vi "Read Profile Data From File.vi"(0 "Profile Data File":path=path "C:/Grabit/Software/VI's/Profiles.ini", 5 "Profile Name":string="Profile1", 11 "error in (no error)":errorcluster) -> (4 "Profile Data":string="0001020304050607080910111213141516171819202122232425262728293031323334353637383940414243444546474849", 15 "error out":errorcluster)   [LabVIEW 2015]
uses:
  <vilib>/Utility/config.llb/Read Key (String).vi
  <vilib>/Utility/config.llb/NI_LVConfig.lvlib
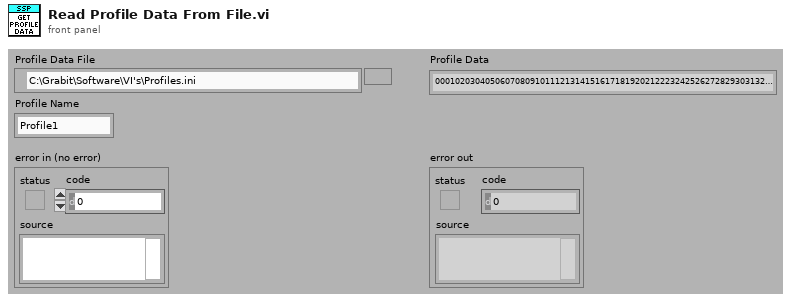
[diagram p1: front panel]
types:
  T1 = typedef "NI_LVConfig.lvlib/Config Data RefNum.ctl" = refnum<k1>
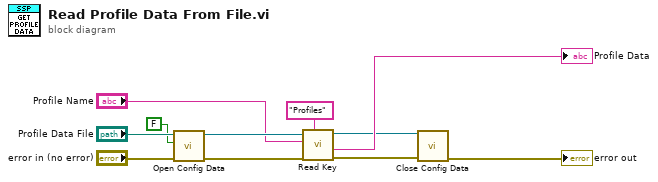
[diagram p0: block diagram]
diagram:
  n1 = call <vilib>:"Open Config Data.vi"("error in (no error)"="error in (no error)", "create file if necessary (T)"=FALSE, "configuration file path"="Profile Data File") -> ("error out"=w10:errorcluster, "refnum"=w11:T1)  [unwired: 6 in, 1 out]
  n2 = call-poly <vilib>:"Read Key.vi"("section"="Profiles", "error in (no error)"=w10, "key"="Profile Name", "refnum"=w11) -> ("error out"=w3:errorcluster, "value"=→"Profile Data":string, "refnum out"=w4:T1)  [unwired: 4 in, 1 out]
  n3 = call <vilib>:"Close Config Data.vi"("error in (no error)"=w3, "refnum"=w4) -> ("error out"=→"error out":errorcluster)  [unwired: 8 in, 1 out]
